vi "Arrayexample.vi"() -> ()   [LabVIEW 2015]
panel:
  out "Matriz 2D":dbl[][](array[numeric])
  out "Matriz 1D\nconcatenacion":dbl[](array[numeric])
  out "Matriz 1D":dbl[](array[numeric])
  in  "stop":bool
  in  "Scalar":dbl
  in  "Array 2":dbl[](array[numeric])
  out "Numeric":dbl
  out "Array":dbl[](array[numeric])
  # "Las matrices te permiten agrupar datos del \nmismo tipo. Una matriz viene determinada por el numero de elementos\ny su dimension. Los elementos son los datos que componen a l a matriz.\nLa dimension es la longitud, altura o profundidad de la matriz\nLabview empieza a contar las matrices desde 0. Y tienen un tamaño maximo\nde pow(2,31) elementos"
  # "No es posible crear una matriz cuyos elementos son una matriz."
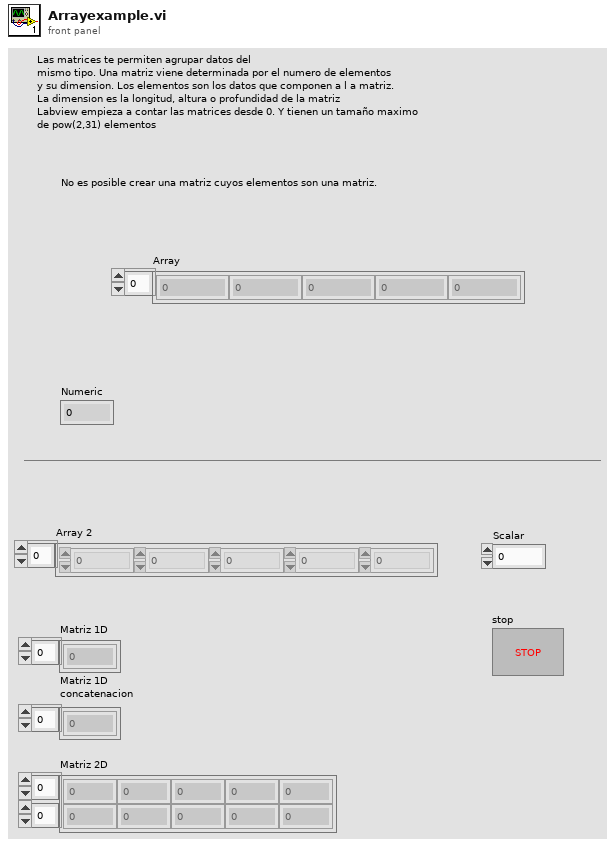
[diagram p1: front panel]
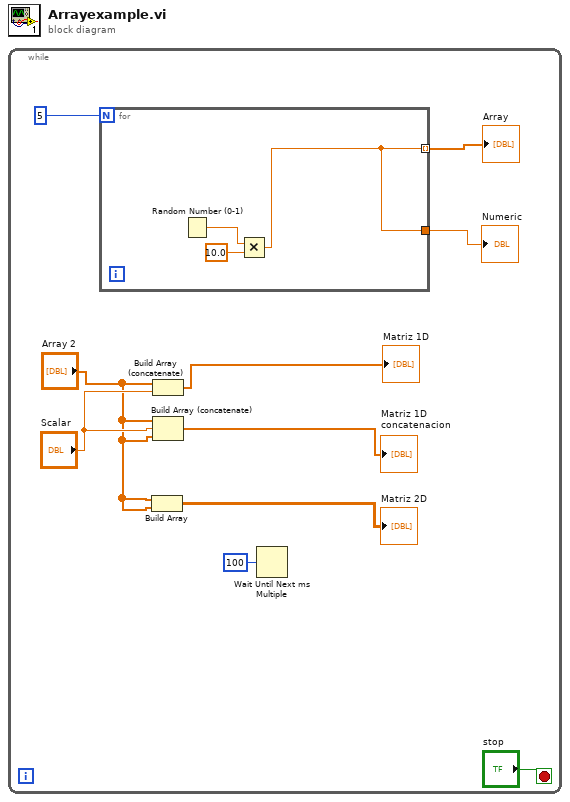
[diagram p0: block diagram]
diagram:
  n1 = while {
    stop <- "stop" stop-if-true
    n2 = for {
      N: 5 -> [_]
      tunnel: [w11] -> w9 mode=indexing
      tunnel: [w11] -> w8
      n3 = Random Number (0-1)() -> (number: 0 to 1=w12:dbl)
      n4 = Multiply(x=w12, y=10.0) -> (x*y=w11:dbl)
    }
    "Array" <- w9
    "Numeric" <- w8
    n5 = Build Array("Array 2", "Array 2") -> (→"Matriz 2D":dbl[][])
    n6 = Build Array (concatenate)("Array 2", "Scalar") -> (→"Matriz 1D":dbl[])
    n7 = Build Array (concatenate)("Array 2", "Scalar", "Array 2") -> (→"Matriz 1D\nconcatenacion":dbl[])
    n8 = Wait Until Next ms Multiple(millisecond multiple=u32 100) -> ()  [unwired: 1 out]
  }
